vi "SCP Wrapper.vi"(6 "Target Directory":string, 7 "Hostname or IP":string, 8 "error in (no error)":errorcluster, 9 "Password":string, 10 "Username":string, 11 "Local Path":path) -> (0 "error out":errorcluster)   [LabVIEW 2019, in "LMH-LINX.lvlib"]
uses:
  <vilib>/MakerHub/LINX/LMH-LINX.lvlib
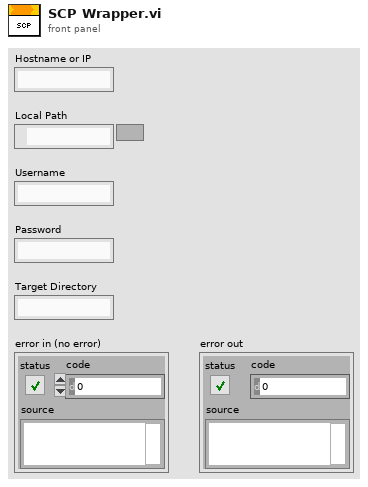
[diagram p1: front panel]
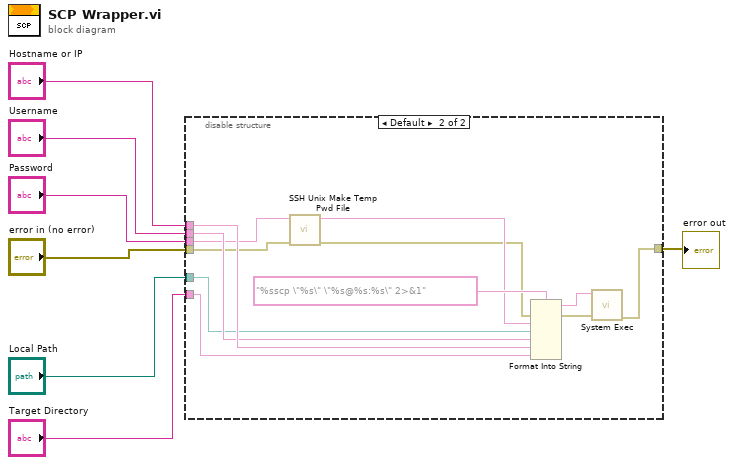
[diagram p0: block diagram]
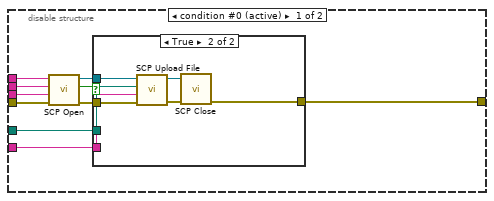
[diagram p2: hidden frame]
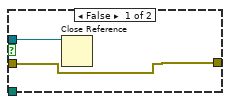
[diagram p3: hidden frame]
diagram:
  n1 = disable-structure shown="Default" {
    disable-tunnel: [w16 w32] -> w7
    disable-tunnel: "Target Directory" -> [w15 w35]
    disable-tunnel: "Local Path" -> [w14 w31]
    disable-tunnel: "Password" -> [w11 w30]
    disable-tunnel: "error in (no error)" -> [w10 w29]
    disable-tunnel: "Username" -> [w9 w36]
    disable-tunnel: "Hostname or IP" -> [w8 w37]
    frame condition #0 (active) {
      n2 = call <vilib>:"SCP Open.vi"("Error In"=w10, "Password"=w11, "Username"=w9, "Hostname or IP"=w8) -> ("Error Out"=w13:errorcluster, "Connected?"=w17:bool, "SCP Session"=w12:refnum<k24>)  [unwired: 5 in]
      n3 = case shown="True" w17 {
        tunnel: w12 -> [w19 w26]
        tunnel: w13 -> [w18 w25]
        tunnel: w14 -> [_ w24]
        tunnel: w15 -> [_ w21]
        tunnel: [w18 w20] -> w16
        frame False {
          n4 = Close Reference(reference=w19) -> ()  [unwired: 1 in, 1 out]
        }
        frame True {
          n5 = call <vilib>:"SCP Upload File.vi"("Error In"=w25, "Target Directory"=w21, "Local File"=w24, "SCP Session"=w26) -> ("Error Out"=w22:errorcluster, "SCP Session"=w23:refnum<k24>)  [unwired: 6 in]
          n6 = call <vilib>:"SCP Close.vi"("Error In"=w22, "SCP Session"=w23) -> ("Error Out"=w20:errorcluster)  [unwired: 9 in]
        }
      }
    }
    frame condition #1 {
      n7 = call <vilib>:"SSH Unix Make Temp Pwd File.vi"("error in (no error)"=w29, "Password"=w30) -> ("error out"=w27:errorcluster, "sshpass command prefix"=w28:string)  [unwired: 8 in]
      n8 = Format Into String(format string="%sscp \"%s\" \"%s@%s:%s\" 2>&1", error in=w27, w28, w31, w36, w37, w35) -> (resulting string=w34:string, error out=w33:errorcluster)  [unwired: 1 in]
      n9 = call <vilib>:"System Exec.vi"("error in (no error)"=w33, "command line"=w34) -> ("error out"=w32:errorcluster)  [unwired: 6 in, 3 out]
    }
  }
  "error out" <- w7
